vi "PathPlanner_PathConstraints_GetAll.vi"(11 "PathPlannerConstraints":T1) -> (0 "MaxAngularAccRadPSecSq":dbl, 1 "MaxAngularVelRadPsEc;":dbl, 2 "MaxAccelerationMpsSq;":dbl, 3 "MaxVelocityMps;":dbl)   [LabVIEW 2019, in "PathPlanner24.lvlib"]
doc: "/**\n * Create a new path constraints object\n *\n * @param maxVelocityMps Max linear velocity (M/S)\n * @param maxAccelerationMpsSq Max linear acceleration (M/S^2)\n * @param maxAngularVelocityRps Max angular velocity (Rad/S)\n * @param maxAngularAccelerationRpsSq Max angular acceleration (Rad/S^2)\n */"
uses:
  PathPlanner24.lvlib
  TypeDef/PathPlannerPathConstraints.ctl
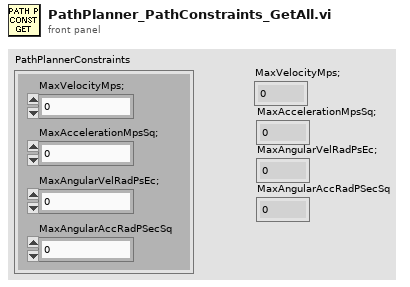
[diagram p1: front panel]
types:
  T1 = typedef "PathPlanner24.lvlib/PathPlannerPathConstraints.ctl" = cluster{"MaxVelocityMps;":dbl, "MaxAccelerationMpsSq;":dbl, "MaxAngularVelRadPsEc;":dbl, "MaxAngularAccRadPSecSq":dbl}
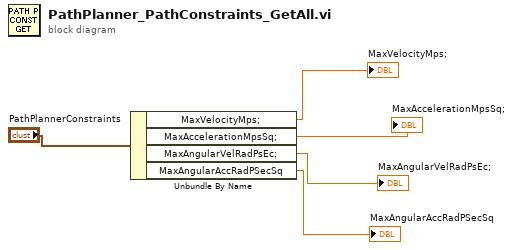
[diagram p0: block diagram]
diagram:
  n1 = Unbundle By Name("PathPlannerConstraints") -> ("MaxVelocityMps;"=→"MaxVelocityMps;":dbl, "MaxAccelerationMpsSq;"=→"MaxAccelerationMpsSq;":dbl, "MaxAngularVelRadPsEc;"=→"MaxAngularVelRadPsEc;":dbl, "MaxAngularAccRadPSecSq"=→"MaxAngularAccRadPSecSq":dbl)
